vi "HH_TraceAndHisto.vi"(0 "Data In":u32[](array[numeric]), 1 "Reset":bool, 5 "Data Count":i32, 11 "Trace Bins":i32=25) -> (4 "Histograms":i32[][](array[numeric]), 6 "Total Photon Count":u64[](array[numeric]), 13 "Total Oveflow Count":u64, 14 "Num Records Total":i64, 15 "Traces":i32[][](array[numeric]))   [LabVIEW 2011]
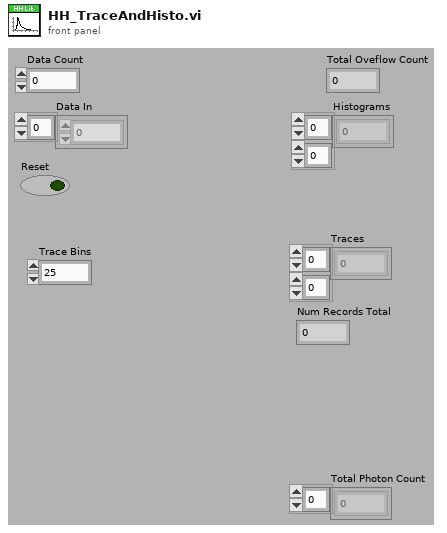
[diagram p1: front panel]
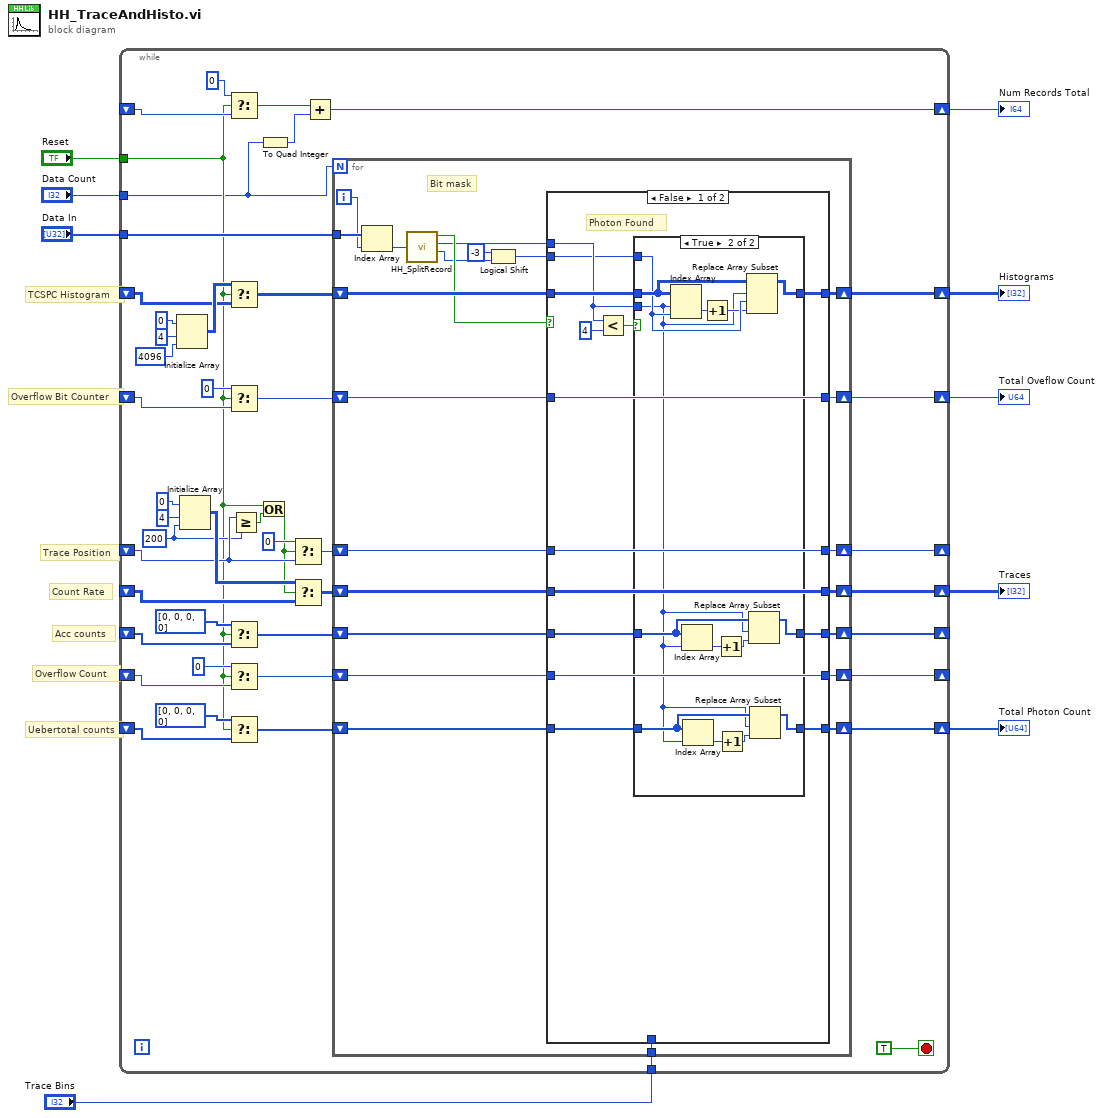
[diagram p0: block diagram]
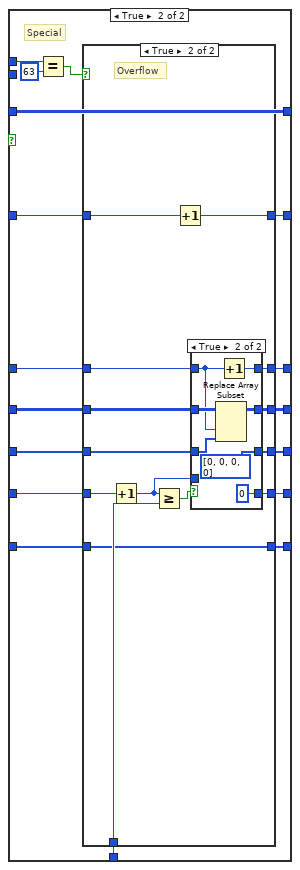
[diagram p3: hidden frame]
diagram:
  # "Uebertotal counts"
  # "Trace Position"
  # "Overflow Count"
  # "Acc counts"
  # "Count Rate"
  # "TCSPC Histogram"
  # "Overflow Bit Counter"
  n1 = while {
    tunnel: "Data In" -> [w53]
    shift-right: [w54] -> w9
    shift-left: _ -> [w49]
    tunnel: "Reset" -> [w12]
    shift-right: [w46] -> w2
    shift-left: _ -> [w45]
    shift-right: [w41] -> w5
    shift-left: _ -> [w40]
    shift-right: [w38] -> _
    shift-left: _ -> [w37]
    shift-right: [w35] -> _
    shift-left: _ -> [w34]
    tunnel: "Trace Bins" -> [w33]
    shift-right: [w30] -> _
    shift-left: _ -> [w28]
    tunnel: "Data Count" -> [w11]
    shift-right: [w23] -> w3
    shift-left: _ -> [w25]
    shift-right: [w14] -> w1
    shift-left: _ -> [w13]
    stop <- TRUE stop-if-true
    w20 = 200 ("dimension size")
    n2 = Initialize Array(0 ("element"), 4 ("dimension size"), 4096 ("dimension size")) -> (w50:i32[][])
    n3 = Initialize Array(0 ("element"), 4 ("dimension size"), w20) -> (w43:i32[][])
    n4 = Select(t=i64 0 ("Data Count 2"), s=w12, f=w25) -> (s? t:f=w24:i64)
    n5 = Select(t=w50, s=w12, f=w49) -> (s? t:f=w51:i32[][])
    n6 = Select(t=u64 0, s=w12, f=w45) -> (s? t:f=w47:u64)
    n7 = Select(t=u32[] [0, 0, 0, 0] ("initialized array"), s=w12, f=w37) -> (s? t:f=w39:u32[])
    n8 = Select(t=u32 0, s=w12, f=w34) -> (s? t:f=w36:u32)
    n9 = Select(t=u64[] [0, 0, 0, 0] ("initialized array"), s=w12, f=w13) -> (s? t:f=w15:u64[])
    n10 = Greater Or Equal?(x=w28, y=w20) -> (x >= y?=w29:bool)
    n11 = Or(x=w12, y=w29) -> (x .or. y?=w27:bool)
    n12 = To Quad Integer(1:w11) -> (0:w10:i64)
    n13 = Select(t=0, s=w27, f=w28) -> (s? t:f=w31:i32)
    n14 = Select(t=w43, s=w27, f=w40) -> (s? t:f=w42:i32[][])
    n15 = Add(x=w24, y=w10) -> (x+y=w23:i64)
    n16 = for {
      N: w11 -> [_]
      tunnel: w53 -> [w65]
      shift-right: [w77] -> w54
      shift-left: w51 -> [w78]
      shift-right: [w75] -> w46
      shift-left: w47 -> [w76]
      shift-right: [w71] -> w41
      shift-left: w42 -> [w72]
      shift-right: [w73] -> w38
      shift-left: w39 -> [w74]
      shift-right: [w69] -> w35
      shift-left: w36 -> [w70]
      tunnel: w33 -> [w68]
      shift-right: [w66] -> w30
      shift-left: w31 -> [w67]
      shift-right: [w61] -> w14
      shift-left: w15 -> [w62]
      i -> [w64]
      # "Bit mask"
      n17 = Index Array(array=w65, index=w64) -> (element=w63:u32)
      n18 = call "HH_SplitRecord.vi"("Record in"=w63) -> ("Special"=w60:bool, "channel"=w59:i32, "time"=w58:i32)  [unwired: 1 out]
      n19 = Logical Shift(y=i8 -3, x=w58) -> (x << y=w56:i32)
      n20 = case shown="False" w60 {
        tunnel: w78 -> [w92 w124]
        tunnel: w59 -> [w80 w112]
        tunnel: [w91 w124] -> w77
        tunnel: w56 -> [w79 _]
        tunnel: w76 -> [w90 w126]
        tunnel: [w90 w125] -> w75
        tunnel: w74 -> [w86 w122]
        tunnel: [w85 w118] -> w73
        tunnel: w72 -> [w89 w121]
        tunnel: [w89 w117] -> w71
        tunnel: w70 -> [w88 w123]
        tunnel: [w88 w119] -> w69
        tunnel: w68 -> [_ w120]
        tunnel: w67 -> [w87 w116]
        tunnel: [w87 w115] -> w66
        tunnel: w62 -> [w82 w114]
        tunnel: [w81 w113] -> w61
        frame False {
          # "Photon Found"
          n21 = Less?(x=w80, y=4) -> (x < y?=w84:bool)
          n22 = case shown="True" w84 {
            tunnel: w92 -> [w95 w109]
            tunnel: [w95 w108] -> w91
            tunnel: w79 -> [_ w107]
            tunnel: w80 -> [_ w96]
            tunnel: w86 -> [w94 w106]
            tunnel: [w94 w105] -> w85
            tunnel: w82 -> [w93 w98]
            tunnel: [w93 w97] -> w81
            frame False {
            }
            frame True {
              n23 = Index Array(array=w109, index (row)=w96, index (col)=w107) -> (element=w104:i32)
              n24 = Index Array(array=w106, index=w96) -> (element=w102:u32)
              n25 = Index Array(array=w98, index=w96) -> (element=w100:u64)
              n26 = Increment(x=w104) -> (x+1=w103:i32)
              n27 = Increment(x=w102) -> (x+1=w101:u32)
              n28 = Increment(x=w100) -> (x+1=w99:u64)
              n29 = Replace Array Subset(array=w109, new element=w103, index (row)=w96, index (col)=w107) -> (w108:i32[][])
              n30 = Replace Array Subset(array=w106, new element=w101, index=w96) -> (w105:u32[])
              n31 = Replace Array Subset(array=w98, new element=w99, index=w96) -> (w97:u64[])
            }
          }
        }
        frame True {
          # "Special"
          n32 = Equal?(x=w112, y=63) -> (x = y?=w110:bool)
          n33 = case shown="True" w110 {
            tunnel: w126 -> [w132 w146]
            tunnel: [w132 w145] -> w125
            tunnel: w123 -> [w131 w135]
            tunnel: w122 -> [w130 w141]
            tunnel: w121 -> [w129 w139]
            tunnel: w120 -> [_ w144]
            tunnel: [w131 w142] -> w119
            tunnel: [w130 w140] -> w118
            tunnel: [w129 w138] -> w117
            tunnel: w116 -> [w128 w137]
            tunnel: [w128 w136] -> w115
            tunnel: w114 -> [w127 w133]
            tunnel: [w127 w133] -> w113
            frame False {
              # "Trigger Signal"
            }
            frame True {
              # "Overflow"
              n34 = Increment(x=w135) -> (x+1=w134:u32)
              n35 = Greater Or Equal?(x=w134, y=w144) -> (x >= y?=w143:bool)
              n36 = Increment(x=w146) -> (x+1=w145:u64)
              n37 = case shown="True" w143 {
                tunnel: w134 -> [w150 _]
                tunnel: [w150 u32 0] -> w142
                tunnel: w141 -> [w149 w155]
                tunnel: [w149 u32[] [0, 0, 0, 0] ("initialized array")] -> w140
                tunnel: w139 -> [w148 w156]
                tunnel: [w148 w154] -> w138
                tunnel: w137 -> [w147 w152]
                tunnel: [w147 w153] -> w136
                frame False {
                }
                frame True {
                  n38 = Replace Array Subset(array=w156, new element=w155, index (col)=w152) -> (w154:i32[][])  [unwired: 1 in]
                  n39 = Increment(x=w152) -> (x+1=w153:i32)
                }
              }
            }
          }
        }
      }
    }
  }
  "Histograms" <- w9
  "Traces" <- w5
  "Num Records Total" <- w3
  "Total Oveflow Count" <- w2
  "Total Photon Count" <- w1
